vi "Get Alias Endpoint.vi"(8 "error in":errorcluster, 10 "alias":string, 11 "endpoint aliases in":T2 format="%.0x") -> (0 "error out":errorcluster, 2 "endpoint":T1, 3 "endpoint aliases out":T2 format="%.0x")   [LabVIEW 2020, in "Routing and Faulting Scripting.lvlib"]
doc: "Returns the endpoint of a specified alias."
uses:
  Routing and Faulting Scripting.lvlib
  <vilib>/NI VeriStand/Custom Device API/Custom Device Item Ref.ctl
  Shared/Alias Endpoint.ctl
  <vilib>/NI VeriStand/Custom Device API/Get Item Property (String).vi
  <vilib>/regexp/Match Regular Expression.xnode
  <vilib>/NI VeriStand/Custom Device API/Custom Device API.lvlib
  Shared/Routing and Faulting Shared.lvlib
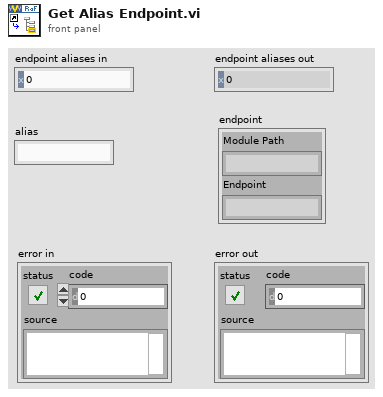
[diagram p1: front panel]
types:
  T1 = typedef "Routing and Faulting Shared.lvlib/Alias Endpoint.ctl" = cluster{"Module Path":string, "Endpoint":string}
  T2 = typedef "Custom Device API.lvlib/Custom Device Item Ref.ctl" = u64
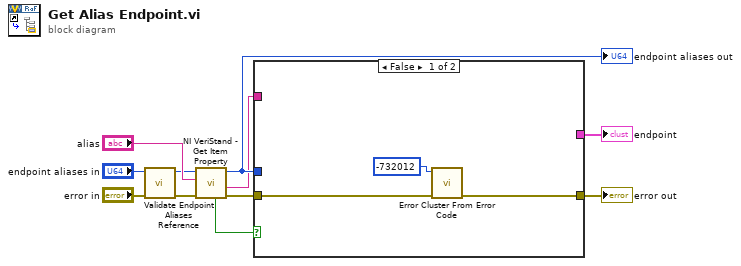
[diagram p0: block diagram]
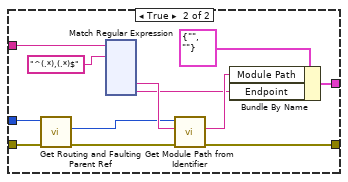
[diagram p2: hidden frame]
diagram:
  n1 = call "Validate Endpoint Aliases Reference.vi"("error in"="error in", "endpoint aliases in"="endpoint aliases in") -> ("error out"=w8:errorcluster, "endpoint aliases out"=w6:T2)  [unwired: 8 in]
  n2 = call-poly <vilib>:"NI VeriStand - Get Item Property.vi"("error in (no error)"=w8, "Property Name"="alias", "Item Ref in"=w6) -> ("error out"=w4:errorcluster, "Value"=w2:string, "Item Ref out"=w3:T2, "Found?"=w10:bool)  [unwired: 5 in]
  "endpoint aliases out" <- w3
  n3 = case shown="False" w10 {
    tunnel: [w13 w17] -> w9
    tunnel: w4 -> [w12 w26]
    tunnel: w3 -> [_ w25]
    tunnel: w2 -> [_ w22]
    tunnel: [_ w16] -> w1
    frame False {
      n4 = call <vilib>:"Error Cluster From Error Code.vi"("error in (no error)"=w12, "error code (0)"=-732012) -> ("error out"=w13:errorcluster)  [unwired: 7 in]
    }
    frame True {
      n5 = call "Get Routing and Faulting Parent Ref.vi"("error in"=w26, "routing and faulting child in"=w25) -> ("error out"=w24:errorcluster, "routing and faulting"=w15:T2)  [unwired: 7 in, 1 out]
      n6 = xnode "Match Regular Expression"("input string"=w22, "regular expression"="^(.*),(.*)$" ("search string")) -> ("submatch 1"=w21:string, "submatch 2"=w18:string)  [unwired: 4 in, 5 out]
      n7 = call "Get Module Path from Identifier.vi"("error in"=w24, "module identifier"=w21, "routing and faulting in"=w15) -> ("error out"=w17:errorcluster, "module path"=w19:string)  [unwired: 6 in, 1 out]
      n8 = Bundle By Name(cluster=T1 {"Module Path"="", "Endpoint"=""} ("Alias Endpoint"), "Module Path"=w19, "Endpoint"=w18) -> (w16:T1)
    }
  }
  "error out" <- w9
  "endpoint" <- w1
